vi "FlatToRichcif_Template_Status.vi"(5 "OutputClusterType":T1, 11 "InputCluster":T2) -> (3 "OutputCluster":T1)   [LabVIEW 2021, in "Template_client.lvlib"]
uses:
  Template_client.lvlib
  cif_Template_Status_Flat.ctl
  cif_Template_Status.ctl
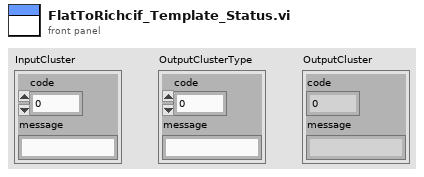
[diagram p1: front panel]
types:
  T1 = typedef "Template_client.lvlib/cif_Template_Status.ctl" = cluster{"code":i32, "message":string}
  T2 = typedef "Template_client.lvlib/cif_Template_Status_Flat.ctl" = cluster{"code":i32, "message":string}
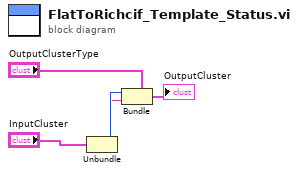
[diagram p0: block diagram]
diagram:
  n1 = Unbundle "Unbundle"("InputCluster") -> ("code"=w2:i32, "message"=w1:string)
  n2 = Bundle "Bundle"(cluster="OutputClusterType", "code"=w2, "message"=w1) -> (→"OutputCluster":T1)
